vi "Random.vi"(12 "Min(0)":dbl format="%#_13g", 14 "Max":dbl format="%#_13g") -> (2 "Random":dbl)   [LabVIEW 2015]
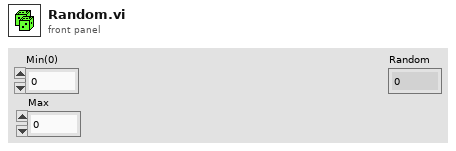
[diagram p1: front panel]
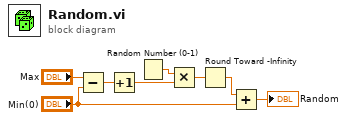
[diagram p0: block diagram]
diagram:
  n1 = Subtract(x="Max", y="Min(0)") -> (x-y=w4:dbl)
  n2 = Increment(x=w4) -> (x+1=w6:dbl)
  n3 = Random Number (0-1)() -> (number: 0 to 1=w8:dbl)
  n4 = Multiply(x=w8, y=w6) -> (x*y=w7:dbl)
  n5 = Round Toward -Infinity(1:w7) -> (0:w3:dbl)
  n6 = Add(x=w3, y="Min(0)") -> (x+y=→"Random":dbl)
